vi "modelParametersFGV.vi"(0 "timeout (-1)":i32=-1) -> (4 "cpu/gpu out":enum32{"Item 0", "Item 1"}(radio)=enum."Item 1", 5 "model out":path caption="Model Path", 6 "classes out":path caption="Class Definition Path", 7 "model params out":T1={"conf"=0.25, "iou"=0.5, "model w"=1280, "model h"=736, "img w "=1280, "img h"=736} caption="Model Parameters")   [LabVIEW 2024]
uses:
  toolkit/modelParameters.ctl
  toolkit/transformCv.lvclass
panel:
  in  "discard":bool
  in  "accept":bool
  in  "cpu/gpu":enum32{"Item 0", "Item 1"}(radio)=enum."Item 1"
  in  "model params":T1={"conf"=0.25, "iou"=0.5, "model w"=1280, "model h"=736, "img w "=1280, "img h"=736} caption="Model Parameters"
  in  "classes":path caption="Class Definition Path"
  in  "model":path caption="Model Path"
  # "Model Parameters"
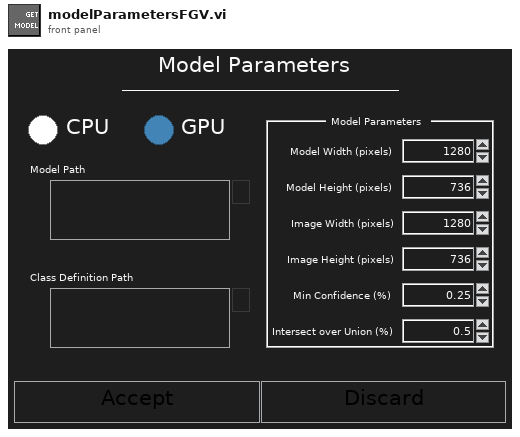
[diagram p1: front panel]
types:
  T1 = typedef "transformCv.lvclass/modelParameters.ctl" = cluster{"conf":dbl, "iou":dbl, "model w":i32, "model h":i32, "img w ":i32, "img h":i32}
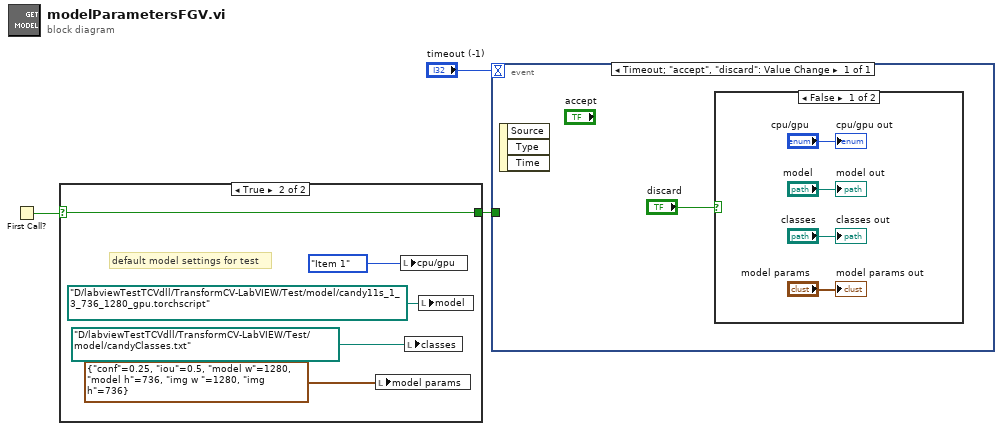
[diagram p0: block diagram]
diagram:
  n1 = First Call?() -> (First Call?: T/F=w2:bool)
  n2 = case shown="True" w2 {
    selector: w2 -> [_ w4]
    tunnel: [_ w4] -> w1
    frame False {
    }
    frame True {
      # "default model settings for test"
      n3 = local write "model params"(T1 {"conf"=0.25, "iou"=0.5, "model w"=1280, "model h"=736, "img w "=1280, "img h"=736} ("model params")) -> ()
      n4 = local write "cpu/gpu"(enum32{"Item 0", "Item 1"}."Item 1" ("cpu/gpu")) -> ()
      n5 = local write "classes"(path "D:/labviewTestTCVdll/TransformCV-LabVIEW/Test/model/candyClasses.txt" ("model")) -> ()
      n6 = local write "model"(path "D:/labviewTestTCVdll/TransformCV-LabVIEW/Test/model/candy11s_1_3_736_1280_gpu.torchscript" ("model")) -> ()
    }
  }
  n7 = event shown="[0] Timeout;  \"accept\", \"discard\": Value Change" {
    selector: _ -> [_]
    dyn-events: _ -> [_]
    timeout: "timeout (-1)" -> [_]
    tunnel: w1 -> [_]
    event Timeout; "accept", "discard": Value Change {
      n8 = event-data() -> ()  [unwired: 1 in, 3 out]
      n9 = case shown="False" "discard" {
        frame False {
          "cpu/gpu out" <- "cpu/gpu"
          "model out" <- "model"
          "classes out" <- "classes"
          "model params out" <- "model params"
        }
        frame True {
        }
      }
    }
  }
